vi "WF3144 4Ch Resistance Output.vi"(2 "Packets (2)":u64[](array[numeric])=[0, 0], 4 "WF3144 I/O":T1={"RES 0"="WF 3144/CH0", "RES 1"="WF 3144/CH1", "RES 2"="WF 3144/CH2", "RES 3"="WF 3144/CH3"}) -> ()   [LabVIEW 2010]
doc: "This VI should be used together with the WF-3144 when creating a custom FPGA for VeriStand.\nIt uses two (2) packets"
uses:
  <vilib>/eio/EIONode/EIONode.xnode
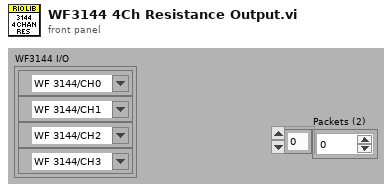
[diagram p1: front panel]
types:
  T1 = cluster{"RES 0":refnum<k21>, "RES 1":refnum<k21>, "RES 2":refnum<k21>, "RES 3":refnum<k21>}
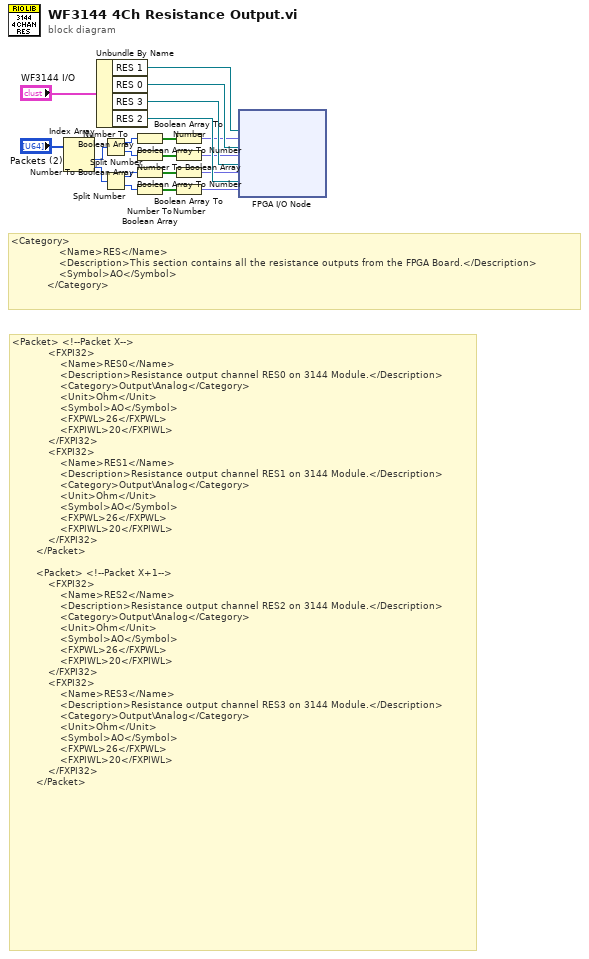
[diagram p0: block diagram]
diagram:
  # "<Category>\n                <Name>RES</Name>\n                <Description>This section contains all the resistance outputs from the FPGA Board.</Description>\n                <Symbol>AO</Symbol>\n            </Category>"
  # "<Packet>\t<!--Packet X-->\n            <FXPI32>\n                <Name>RES0</Name>\n                <Description>Resistance output channel RES0 on 3144 Module.</Description>\n                <Category>Output\\Analog</Category>\n                <Unit>Ohm</Unit>\n                <Symbol>AO</Symbol>\n                <FXPWL>26</FXPWL>\n                <FXPIWL>20</FXPIWL>\n            </FXPI32>\n            <FXPI32>\n                <Name>RES1</Name>\n                <Description>Resistance output channel RES1 on 3144 Module.</Description>\n                <Category>Output\\Analog</Category>\n                <Unit>Ohm</Unit>\n                <Symbol>AO</Symbol>\n                <FXPWL>26</FXPWL>\n                <FXPIWL>20</FXPIWL>\n            </FXPI32>\n        </Packet>\n\t\t\n        <Packet>\t<!--Packet X+1-->\n            <FXPI32>\n                <Name>RES2</Name>\n                <Description>Resistance output channel RES2 on 3144 Module.</Description>\n                <Category>Output\\Analog</Category>\n                <Unit>Ohm</Unit>\n                <Symbol>AO</Symbol>\n                <FXPWL>26</FXPWL>\n                <FXPIWL>20</FXPIWL>\n            </FXPI32>\n            <FXPI32>\n                <Name>RES3</Name>\n                <Description>Resistance output channel RES3 on 3144 Module.</Description>\n                <Category>Output\\Analog</Category>\n                <Unit>Ohm</Unit>\n                <Symbol>AO</Symbol>\n                <FXPWL>26</FXPWL>\n                <FXPIWL>20</FXPIWL>\n            </FXPI32>\n        </Packet>"
  n1 = Index Array(array="Packets (2)") -> (element #1=w2:u64, element #2=w3:u64)  [unwired: 2 in]
  n2 = Unbundle By Name("WF3144 I/O") -> ("RES 1"=w19:refnum<k21>, "RES 0"=w20:refnum<k21>, "RES 3"=w18:refnum<k21>, "RES 2"=w17:refnum<k21>)
  n3 = Split Number(x=w2) -> (hi(x)=w4:u32, lo(x)=w5:u32)
  n4 = Split Number(x=w3) -> (hi(x)=w6:u32, lo(x)=w7:u32)
  n5 = Number To Boolean Array(number=w4) -> (Boolean array=w9:bool[])
  n6 = Number To Boolean Array(number=w5) -> (Boolean array=w11:bool[])
  n7 = Number To Boolean Array(number=w6) -> (Boolean array=w12:bool[])
  n8 = Number To Boolean Array(number=w7) -> (Boolean array=w14:bool[])
  n9 = Boolean Array To Number(Boolean array=w9) -> (number=w8:fxp<+/-,26,20>)
  n10 = Boolean Array To Number(Boolean array=w11) -> (number=w10:fxp<+/-,26,20>)
  n11 = Boolean Array To Number(Boolean array=w12) -> (number=w13:fxp<+/-,26,20>)
  n12 = Boolean Array To Number(Boolean array=w14) -> (number=w15:fxp<+/-,26,20>)
  n13 = xnode "FPGA I/O Node"("I/O Item"=w8, "FPGA I/O In"=w19, "I/O Item"=w10, "FPGA I/O In"=w20, "I/O Item"=w13, "FPGA I/O In"=w18, "I/O Item"=w15, "FPGA I/O In"=w17) -> ()  [unwired: 4 out]
